vi "SMTPSimple.vi"(8 "错误输入（无错误）":errorcluster, 9 "body":string, 11 "messenger":T1={"host"="smtp-mail.outlook.com", "port"=587, "username"="", "password"="", "From"="", "to"="", "subject"="", "postURL"=""}) -> (0 "error out":errorcluster)   [LabVIEW 2017]
panel:
  in  "IsBodyHtml":bool=TRUE
  in  "EnableSSl":bool=TRUE
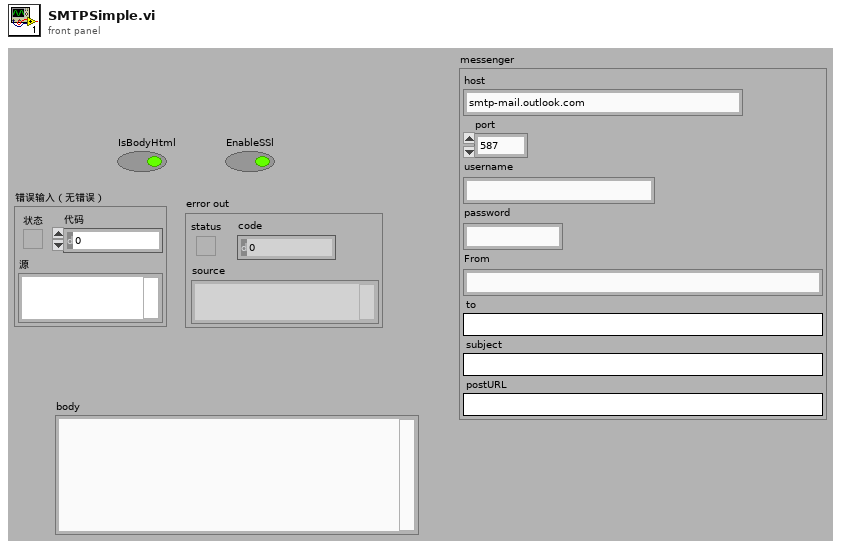
[diagram p1: front panel]
types:
  T1 = cluster{"host":string, "port":i32, "username":string, "password":string, "From":string, "to":string, "subject":string, "postURL":string}
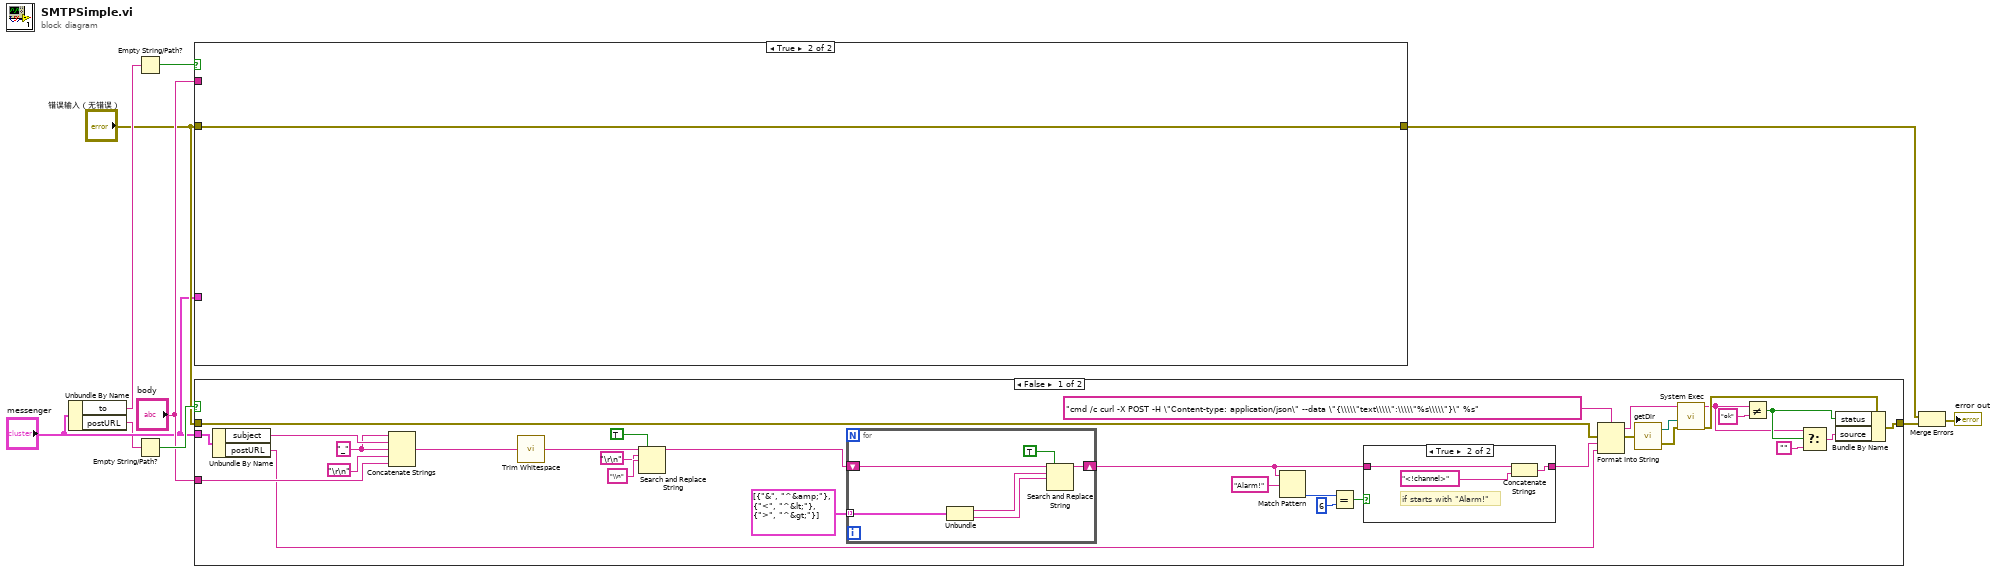
[diagram p0: block diagram]
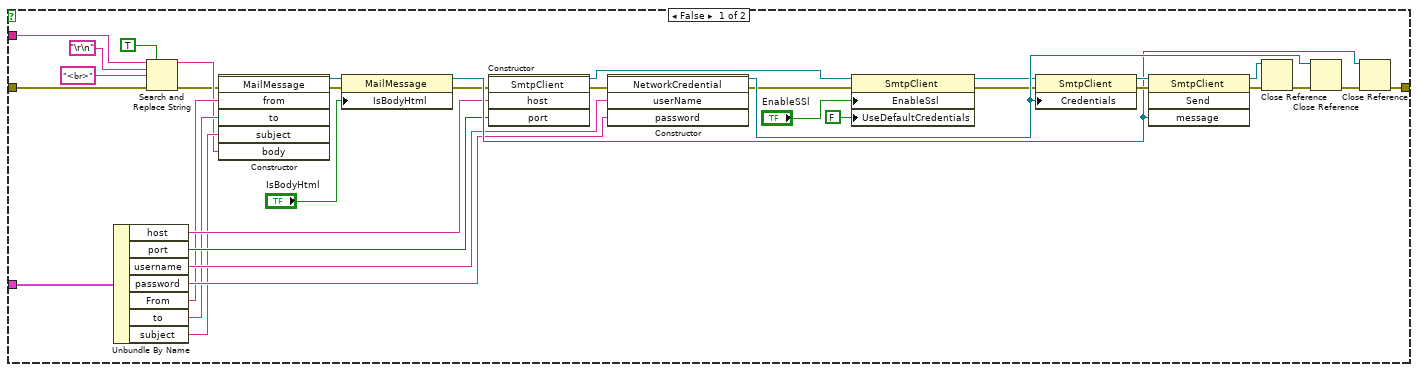
[diagram p4: hidden frame]
diagram:
  n1 = Unbundle By Name("messenger") -> ("to"=w8:string, "postURL"=w1:string)
  n2 = Empty String/Path?(string/path=w8) -> (empty?=w7:bool)
  n3 = Empty String/Path?(string/path=w1) -> (empty?=w6:bool)
  n4 = case shown="True" w7 {
    tunnel: "messenger" -> [w19 _]
    tunnel: "错误输入（无错误）" -> [w13 w46]
    tunnel: [w18 w46] -> w3
    tunnel: "body" -> [w11 _]
    frame False {
      n5 = Unbundle By Name(w19) -> ("host"=w26:string, "port"=w25:i32, "username"=w24:string, "password"=w23:string, "From"=w22:string, "to"=w21:string, "subject"=w20:string)
      n6 = Search and Replace String(replace all?=TRUE ("替换全部？(F)"), input string=w11, search string="\r\n", replace string="<br>" ("替换字符串(\"\")"), error in=w13) -> (result string=w15:string, error out=w12:errorcluster)  [unwired: 5 out]
      n7 = constructor class="MailMessage"(error in=w12, "from"=w22, "to"=w21, "subject"=w20, "body"=w15) -> (reference out=w30:refnum<k24>, error out=w28:errorcluster)  [unwired: 2 in, 5 out]
      n8 = property class="MailMessage"(reference=w30, error in=w28, "IsBodyHtml"="IsBodyHtml") -> (reference out=w29:refnum<k24>, error out=w27:errorcluster)
      n9 = constructor class="SmtpClient"(error in=w27, "host"=w26, "port"=w25) -> (reference out=w38:refnum<k24>, error out=w40:errorcluster)  [unwired: 2 in, 3 out]
      n10 = constructor class="NetworkCredential"(error in=w40, "userName"=w24, "password"=w23) -> (reference out=w43:refnum<k24>, error out=w39:errorcluster)  [unwired: 2 in, 3 out]
      n11 = property class="SmtpClient"(reference=w38, error in=w39, "EnableSsl"="EnableSSl", "UseDefaultCredentials"=FALSE) -> (reference out=w37:refnum<k24>, error out=w36:errorcluster)
      n12 = property class="SmtpClient"(reference=w37, error in=w36, "Credentials"=w43) -> (reference out=w33:refnum<k24>, error out=w32:errorcluster)
      n13 = invoke class="SmtpClient" method="Send"(reference=w33, error in=w32, "message"=w29) -> (reference out=w35:refnum<k24>, error out=w34:errorcluster)  [unwired: 1 in, 2 out]
      n14 = Close Reference(reference=w35, error in (no error)=w34) -> (error out=w42:errorcluster)
      n15 = Close Reference(reference=w43, error in (no error)=w42) -> (error out=w41:errorcluster)
      n16 = Close Reference(reference=w29, error in (no error)=w41) -> (error out=w18:errorcluster)
    }
    frame True {
    }
  }
  n17 = case shown="False" w6 {
    tunnel: [w73 w89] -> w10
    tunnel: "body" -> [w67 _]
    tunnel: "错误输入（无错误）" -> [w72 w89]
    tunnel: "messenger" -> [w68 _]
    frame False {
      w53 = "_" ("字符串")
      n18 = Unbundle By Name(w68) -> ("subject"=w54:string, "postURL"=w63:string)
      n19 = Concatenate Strings(w53, w54, w53, "\r\n", w67) -> (w59:string)
      n20 = call <vilib>:"Trim Whitespace.vi"("string"=w59) -> ("trimmed string"=w58:string)  [unwired: 1 in]
      n21 = Search and Replace String(replace all?=TRUE ("替换全部？(F)"), input string=w58, search string="\r\n", replace string="\\n" ("替换字符串(\"\")")) -> (result string=w55:string)  [unwired: 1 in, 6 out]
      n22 = for {
        shift-right: [w85] -> w51
        shift-left: w55 -> [w84]
        tunnel: cluster{string, string}[] [{"&", "^&amp;"}, {"<", "^&lt;"}, {">", "^&gt;"}] -> [w88] mode=indexing
        n23 = Unbundle(w88) -> (w87:string, w86:string)
        n24 = Search and Replace String(replace all?=TRUE ("替换全部？(F)"), input string=w84, search string=w87, replace string=w86) -> (result string=w85:string)  [unwired: 1 in, 6 out]
      }
      n25 = Match Pattern(string=w51, regular expression="Alarm!") -> (offset past match=w49:i32)  [unwired: 1 in, 3 out]
      n26 = Equal?(x=w49, y=6) -> (x = y?=w47:bool)
      n27 = case shown="True" w47 {
        tunnel: [w79 w80] -> w52
        tunnel: w51 -> [w79 w82]
        frame False {
        }
        frame True {
          # "if starts with \"Alarm!\""
          n28 = Concatenate Strings(w82, "<!channel>" ("string")) -> (w80:string)
        }
      }
      n29 = Format Into String(format string="cmd /c curl -X POST -H \"Content-type: application/json\" --data \"{\\\\\"text\\\\\":\\\\\"%s\\\\\"}\" %s" ("command line"), error in=w72, w52, w63) -> (resulting string=w62:string, error out=w76:errorcluster)  [unwired: 1 in]
      n30 = call "getDir.vi"("错误输入（无错误）"=w76) -> ("stripped path"=w60:path, "错误输出"=w78:errorcluster)
      n31 = call <vilib>:"System Exec.vi"("error in (no error)"=w78, "working directory"=w60, "command line"=w62) -> ("error out"=w75:errorcluster, "standard output"=w70:string)  [unwired: 3 in, 4 out]
      n32 = Not Equal?(x=w70, y="ok" ("standard output")) -> (x != y?=w71:bool)
      n33 = Select(t=w70, s=w71, f="") -> (s? t:f=w61:string)
      n34 = Bundle By Name(cluster=w75, "status"=w71, "source"=w61) -> (w73:errorcluster)
    }
    frame True {
    }
  }
  n35 = Merge Errors(w3, w10) -> (→"error out":errorcluster)
